vi "Keithley24XX_SR830_PPMS_4Probe_Resistance_Measurement.vi"() -> ()   [LabVIEW 2019]
uses:
  <instrlib>/Stanford Research 830/Public/Data/Read (All Parameters).vi
  <instrlib>/Keithley 24XX/Public/Data/Read (Single Point).vi
  <instrlib>/Keithley 24XX/Keithley 24XX.lvlib
  <instrlib>/Stanford Research 830/Stanford Research 830.lvlib
panel:
  in  "PPMS Temp":dbl
  out "Gate\nVoltage":sgl
  out "Status":sgl
  out "Leakage \nCurrent":sgl
  in  "Temp Vs Time":enum32{"XY Graph", "Waveform (Time)"}(tab)
  out "dup path":path
  in  "<File Name>.txt (Don't add extension)":string
  in  "Data Save Path:":path=path "C:/Users/labpc/Documents/ProbeStation Users Data"
  in  "I_leak vs Vg":enum32{"XY Graph", "Waveform (Time)"}(tab)
  out "I_leak vs Vg : XYGraph":cluster{"Y":dbl[], "Y":dbl[]}[](graph)
  out "I_leak vs Vg : TimeGraph":cluster{dbl, "Current":sgl}[](graph)
  in  "Gate Voltage\nInitial (V)":dbl
  out "Gate Voltage\nTraversal Direction":enum16{"Upward", "Downward"}(ring)
  in  "Series Resistance \n(Apparatus Constant)":dbl=10000000.0
  in  "stop":bool
  out "Max/Min(-) \nGate Voltage (V)":dbl=80.0
  in  "Gate Voltage \nStep Size (V)":dbl=0.1
  in  "High Gate \nVoltage (V)":dbl
  in  "Low Gate \nVoltage (V)":dbl
  out "Compliance\n Level (A)":dbl=0.1
  in  "Theta vs Vg":enum32{"XY Graph", "Waveform (Time)"}(tab)
  out "Theta vs Vg : XYGraph":cluster{"Y":dbl[], "Y":dbl[]}[](graph)
  out "Theta vs Vg : TimeGraph":cluster{dbl, "Theta-Value":dbl}[](graph)
  in  "R vs Vg":enum32{"XY Graph", "Waveform (Time)"}(tab)
  out "Resistance vs Vg : XYGraph":cluster{"Y":dbl[], "Y":dbl[]}[](graph)
  out "R vs Vg : TimeGraph":cluster{dbl, dbl}[](graph)
  in  "Sensitivity (Initial Value)":i16(ring)=17 items=["Auto Gain"=-1, "2 nV/fA"=0, "5 nV/fA"=1, "10 nV/fA"=2, "20 nV/fA"=3, "50 nV/fA"=4, "100 nV/fA"=5, "200 nV/fA"=6, "500 nV/fA"=7, "1 uV/pA"=8, "2 uV/pA"=9, "5 uV/pA"=10, "10 uV/pA"=11, "20 uV/pA"=12, "50 uV/pA"=13, "100 uV/pA"=14, "200 uV/pA"=15, "500 uV/pA"=16, "1 mV/nA"=17, "2 mV/nA"=18, "5 mV/nA"=19, "10 mV/nA"=20, "20 mV/nA"=21, "50 mV/nA"=22, "100 mV/nA"=23, "200 mV/nA"=24, "500 mV/mA"=25, "1 V/uA"=26]
  in  "Dynamic Reserve (-1 = Auto)":i16(ring)=-1 items=["Auto Reserve"=-1, "High Reserve"=0, "Normal"=1, "Low Noise"=2]
  in  "Input Connection (0: Single-Ended Voltage)":u16(ring)=1 items=["Single-Ended Voltage", "Differential Voltage", "1 MOhm Current Gain", "100 MOhm Current Gain"]
  out "Input Coupling (0: AC)":u16(ring) items=["AC", "DC"]
  in  "Time Constant (8: 100ms)":u16(ring)=9 items=["10 us", "30 us", "100 us", "300 us", "1 ms", "3 ms", "10 ms", "30 ms", "100 ms", "300 ms", "1 s", "3 s", "10 s", "30 s", "100 s", "300 s", "1 ks", "3 ks", "10 ks", "30 ks"]
  in  "SR830 VISA resource name":refnum<visa-resource-name>="GPIB0::10::INSTR"
  in  "Trigger Source (0: Internal)":u16(ring) items=["Internal", "External"]
  out "Manual Phase (0 Degree)":dbl
  out "Detection Harmonic Number":dbl=1.0
  out "External Reference Trigger (0: Sine Zero Crossing)":u16(ring) items=["Sine Zero Crossing", "TTL Rising Edge", "TTL Falling Edge"]
  in  "Internal Reference Frequency (1000 Hz)":dbl=17.0
  in  "Reference Source (1: Internal)":u16(ring)=1 items=["External", "Internal"]
  in  "Sine Output Amplitude (V)":dbl=1.0
  in  "Serial Configuration":T1={"Baud Rate"=9600, "Parity"=0, "Data Bits"=8, "Stop Bits"=10, "Flow Control"=0} {"Flow Control" items=["None", "XON/XOFF", "RTS/CTS", "XON/XOFF & RTS/CTS", "DTR/DSR", "XON/XOFF & DTR/DSR"]; "Stop Bits" items=["1.0"=10, "1.5"=15, "2.0"=20]; "Data Bits" items=["7"=7, "8"=8]; "Parity" items=["None", "Odd", "Even", "Mark", "Space"]; "Baud Rate" items=["300"=300, "600"=600, "1200"=1200, "2400"=2400, "4800"=4800, "9600"=9600, "19200"=19200]}
  in  "Keithley24XX VISA resource name":refnum<visa-resource-name>="GPIB0::21::INSTR" caption="Keithley 24XX VISA resource name"
  out "Interal Measurement Time":u32
  # "Lake Shore 336 Temp Contr."
  # "SR830 Lock In Amplifier"
  # "MAKE SURE THE SOURCE METER IS ON TO ENSURE NO UNINTENDED JUMPS. PROGRAM WILL KEEP SOURCE METER ON ONCE RUN."
  # "Keithley 2400 SourceMeter"
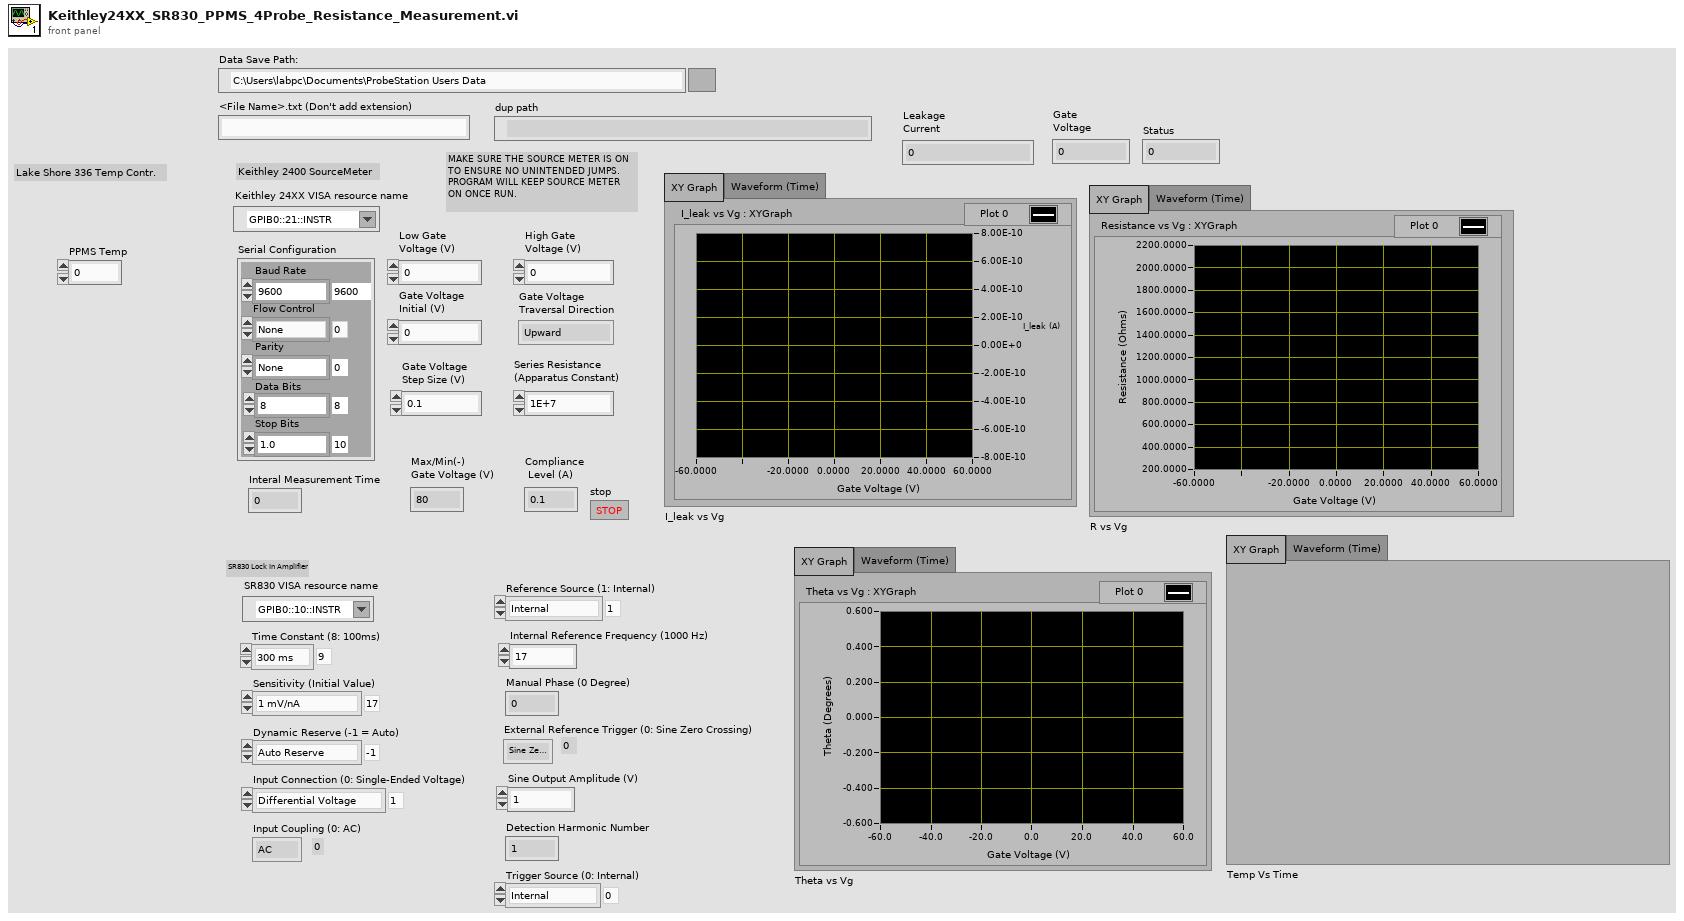
[diagram p1: front panel]
types:
  T1 = cluster{"Baud Rate":u32, "Parity":u16, "Data Bits":u16, "Stop Bits":u16, "Flow Control":u16}
  T2 = enum16{"open", "replace", "create", "open or create", "replace or create", "replace or create with confirmation"}
  T3 = cluster{"X-Value":dbl, "Y-Value":dbl, "R-Value":dbl, "Theta-Value":dbl, "Aux In 1 Value":dbl, "Aux In 2 Value":dbl, "Aux In 3 Value":dbl, "Aux In 4 Value":dbl, "Reference Frequency":dbl, "Channel 1 Display":dbl, "Channel 2 Display":dbl}
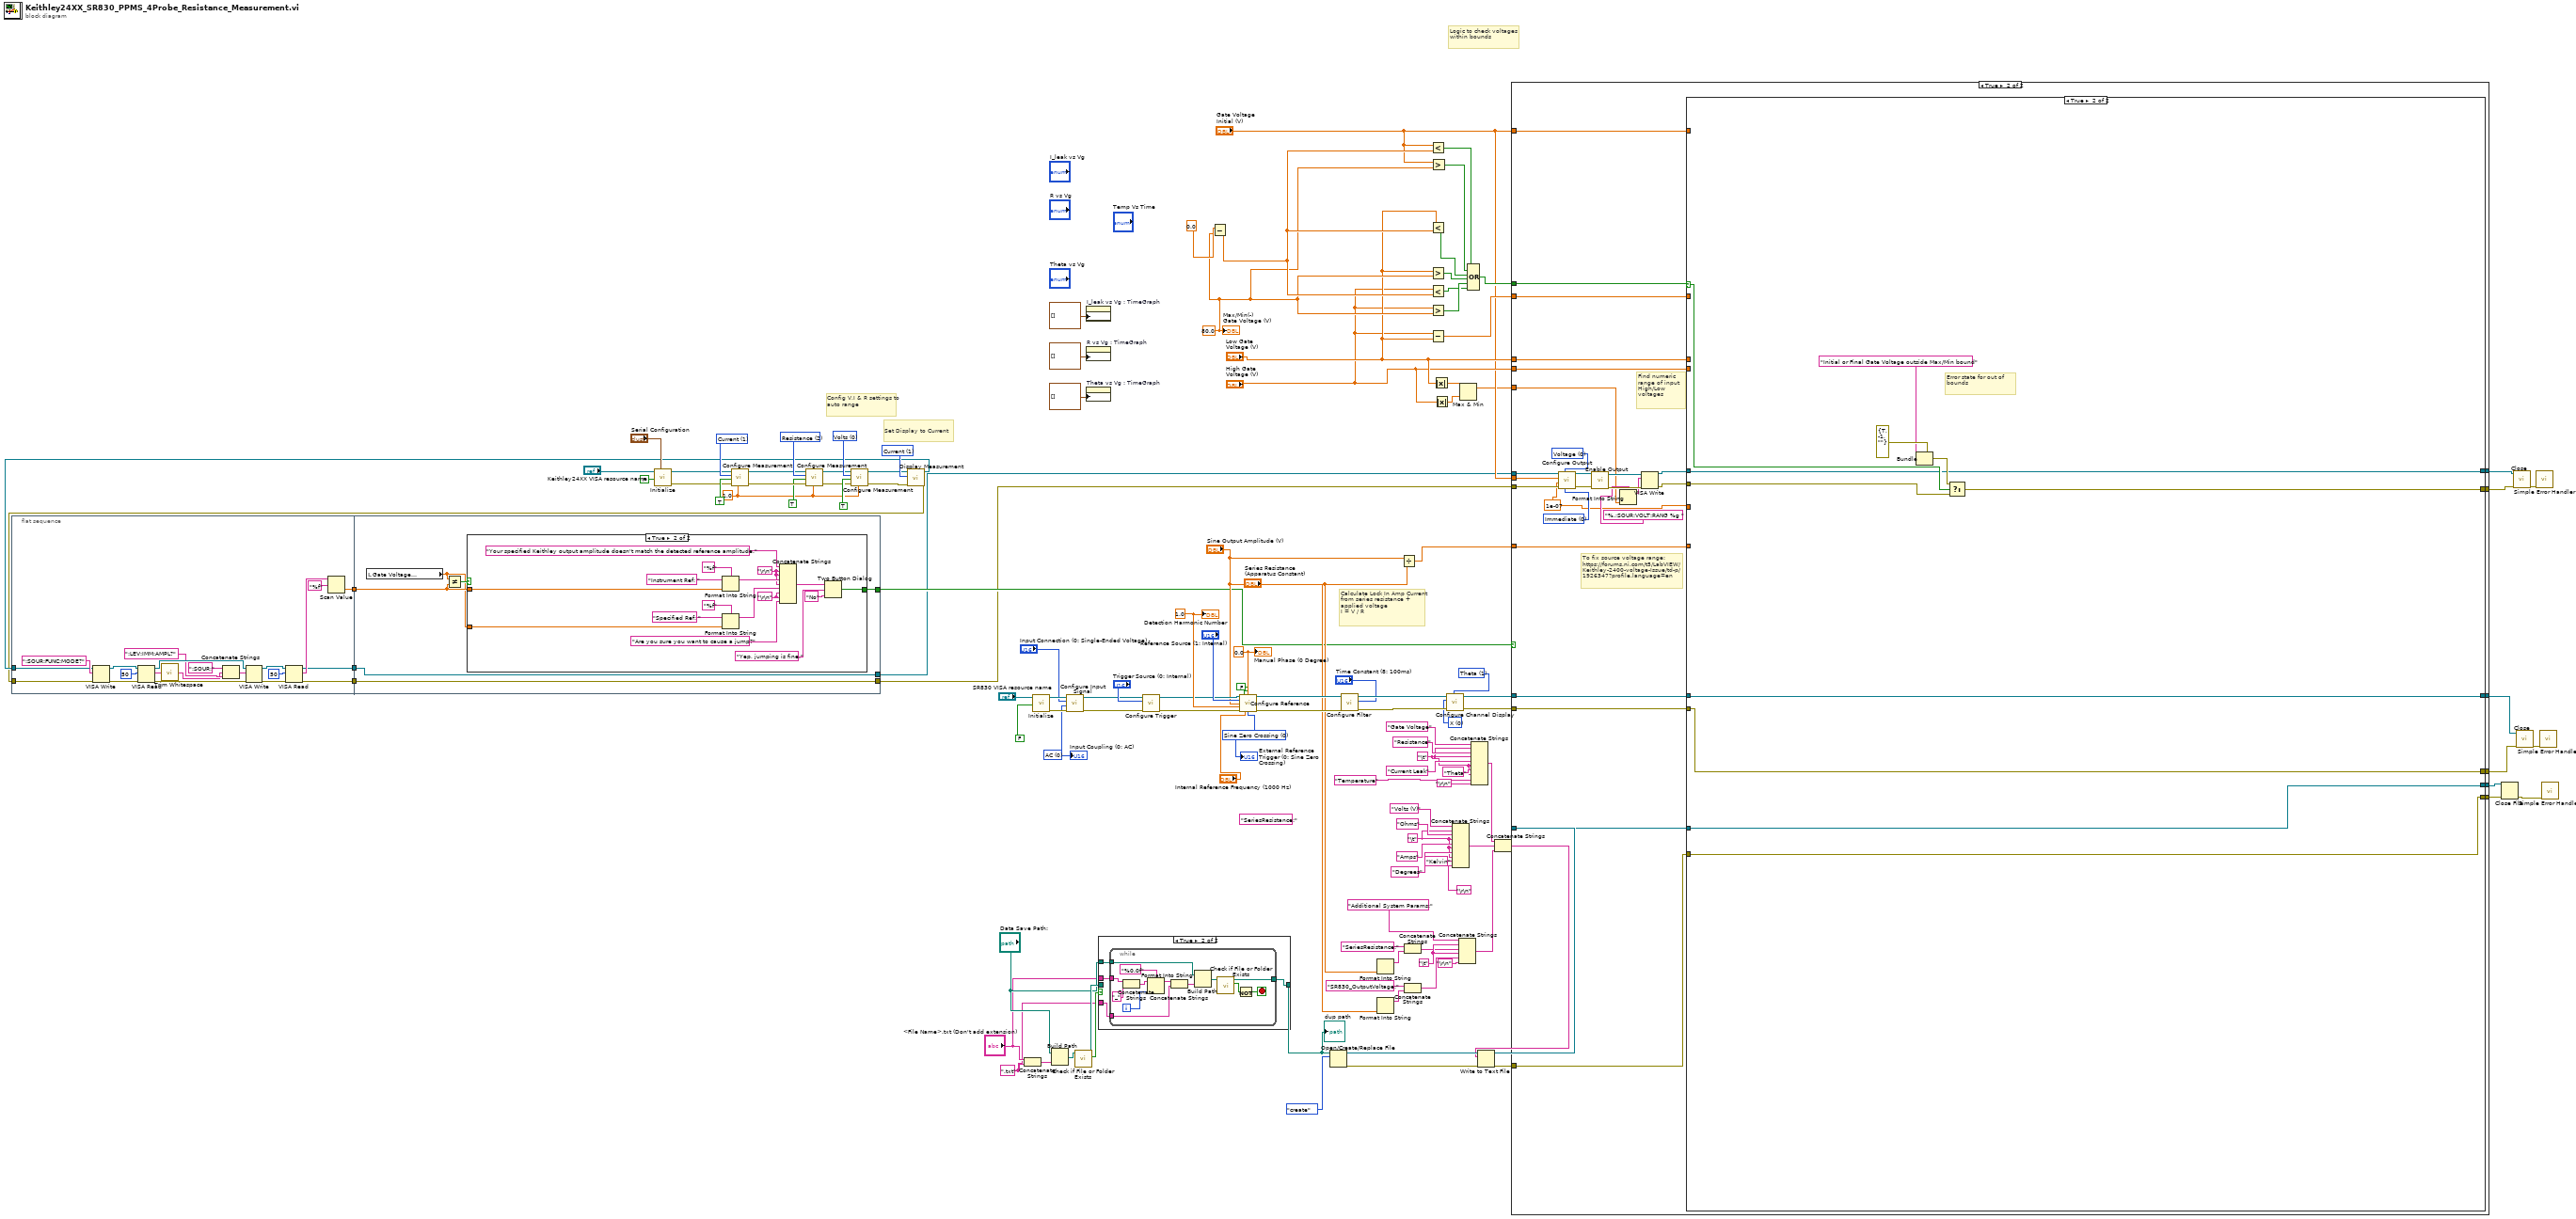
[diagram p0: block diagram]
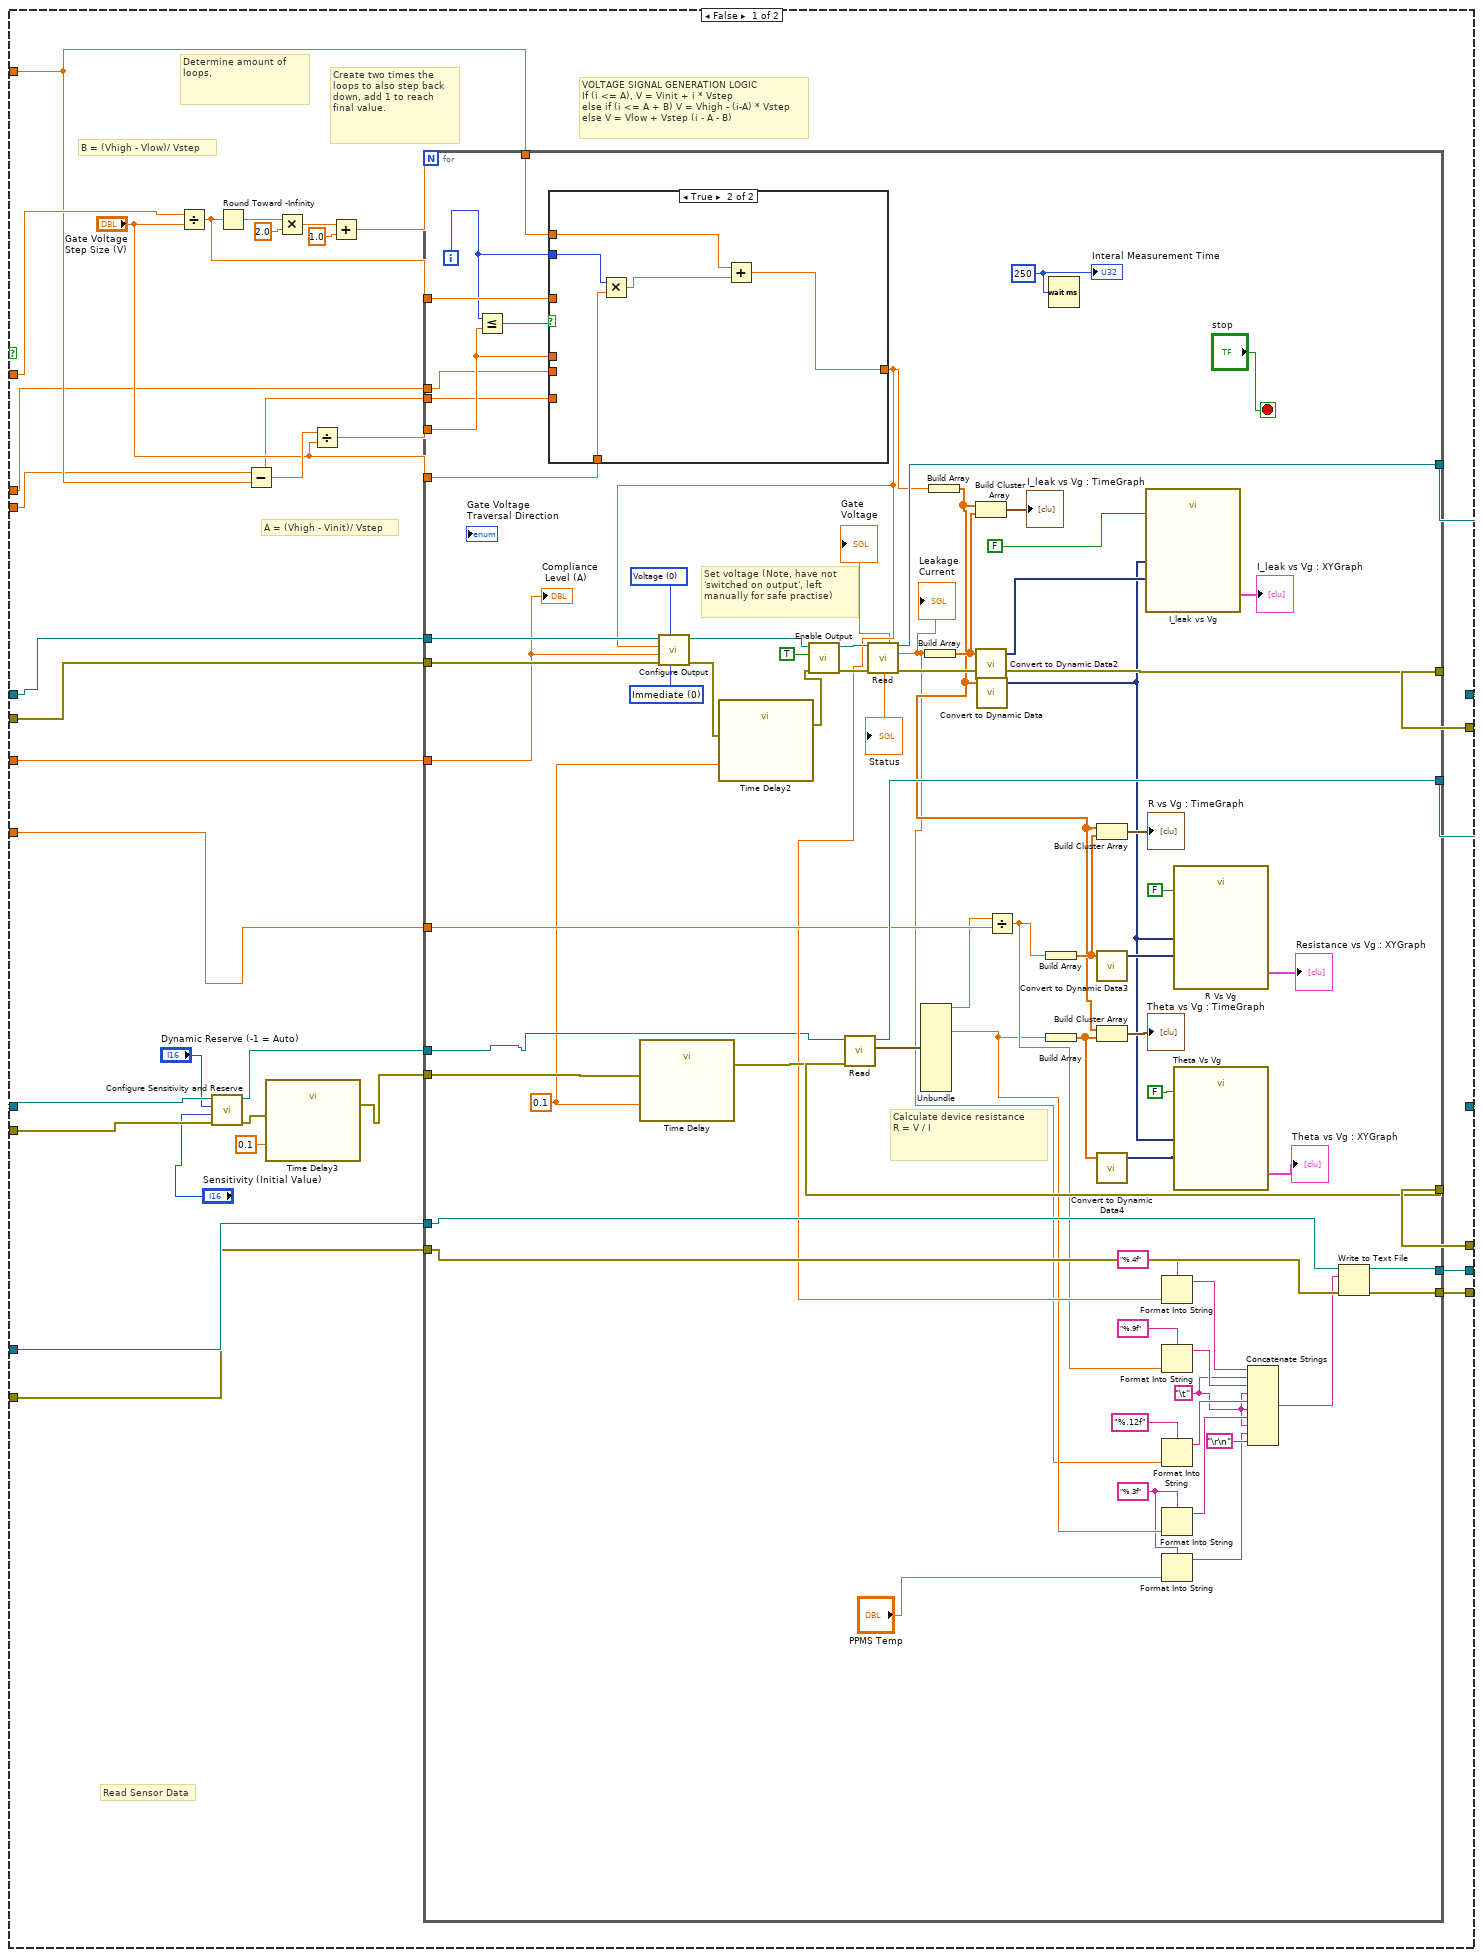
[diagram p3: hidden frame]
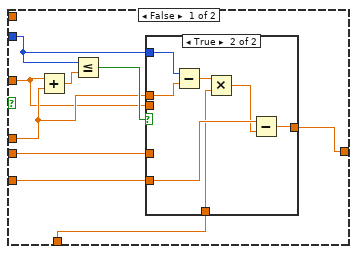
[diagram p4: hidden frame]
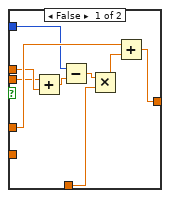
[diagram p5: hidden frame]
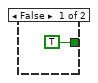
[diagram p6: hidden frame]
diagram:
  w25 = "\t"
  w16 = "\t"
  w18 = "\t"
  (unwired) "SeriesResistance:" ("string")
  w53 = ".txt"
  w60 = 1.0 ("Manual Range (1.0)")
  w84 = 0.0 ("Manual Phase (0 Degree)")
  w85 = 1.0 ("Detection Harmonic Number (1)")
  w86 = u16 0 items=["Sine Zero Crossing", "TTL Rising Edge", "TTL Falling Edge"] ("External Reference Trigger (0: Sine Zero Crossing)")
  w90 = u16 0 items=["AC", "DC"] ("Input Coupling (0: AC)")
  w72 = u16 0 items=["X", "R", "X Noise", "Aux In 1", "Aux In 2"] ("Channel 1 Display (0: X)")
  w100 = u16 1 items=["Y", "Theta", "Y Noise", "Aux In 3", "Aux In 4"] ("Channel 2 Display  (0: Y)")
  w105 = u16 1 items=["Voltage", "Current", "Resistance"] ("Displayed Measurement (0: Voltage)")
  w114 = u16 2 items=["Volts", "Current", "Resistance"] ("Function (0: Volts)")
  w118 = u16 1 items=["Volts", "Current", "Resistance"] ("Function (0: Volts)")
  w61 = 80.0
  w124 = u16 0 items=["Volts", "Current", "Resistance"] ("Function (0: Volts)")
  # "Logic to check voltages within bounds"
  # "Calculate Lock In Amp Current from series resistance + applied voltage\nI = V / R"
  # "Set Display to Current"
  # "Config V,I & R settings to auto range"
  n1 = flat-sequence {
    tunnel: [w128] -> w10
    tunnel: [w129] -> w9
    tunnel: [w130] -> w8
    tunnel: w7 -> [w127]
    tunnel: w6 -> [w126]
    tunnel: w10 -> [w149]
    tunnel: w9 -> [w148]
    tunnel: w8 -> [w152]
    tunnel: [w149] -> w2
    tunnel: [w148] -> w4
    tunnel: [w147] -> w5
    frame #0 {
      n2 = VISA Write(VISA resource name=w127, write buffer=":SOUR:FUNC:MODE?", error in (no error)=w126) -> (VISA resource name out=w143:refnum<visa-resource-name>, error out=w146:errorcluster)  [unwired: 1 out]
      n3 = VISA Read(VISA resource name=w143, byte count=u32 50, error in (no error)=w146) -> (VISA resource name out=w138:refnum<visa-resource-name>, read buffer=w132:string, error out=w139:errorcluster)  [unwired: 1 out]
      n4 = call <vilib>:"Trim Whitespace.vi"("string"=w132) -> ("trimmed string"=w131:string)  [unwired: 1 in]
      n5 = Concatenate Strings(":SOUR:" ("string"), w131, ":LEV:IMM:AMPL?" ("string")) -> (w135:string)
      n6 = VISA Write(VISA resource name=w138, write buffer=w135, error in (no error)=w139) -> (VISA resource name out=w140:refnum<visa-resource-name>, error out=w142:errorcluster)  [unwired: 1 out]
      n7 = VISA Read(VISA resource name=w140, byte count=u32 50, error in (no error)=w142) -> (VISA resource name out=w128:refnum<visa-resource-name>, read buffer=w133:string, error out=w129:errorcluster)  [unwired: 1 out]
      n8 = Scan Value(string=w133, format string="%f") -> (value=w130:dbl)  [unwired: 1 in, 1 out]
    }
    frame #1 {
      n9 = local read "Gate Voltage\nInitial (V)"() -> (w150:dbl)
      n10 = Not Equal?(x=w150, y=w152) -> (x != y?=w151:bool)
      n11 = case shown="True" w151 {
        tunnel: [TRUE ("T button?") w160] -> w147
        tunnel: w152 -> [_ w155]
        tunnel: w150 -> [_ w154]
        frame False {
        }
        frame True {
          w158 = "\r\n"
          w156 = "\r\n"
          n12 = Format Into String(format string="%f", initial string="Instrument Ref: ", w155) -> (resulting string=w162:string)  [unwired: 1 in, 1 out]
          n13 = Format Into String(format string="%f", initial string="Specified Ref: ", w154) -> (resulting string=w161:string)  [unwired: 1 in, 1 out]
          n14 = Concatenate Strings("Your specified Keithley output amplitude doesn't match the detected reference amplitude." ("message"), w156, w156, w162, w156, w161, w158, w158, "Are you sure you want to cause a jump?" ("string")) -> (w167:string)
          n15 = Two Button Dialog(message=w167, 1:"No" ("F button name (\"Cancel\")"), 2:"Yep, jumping is fine." ("T button name (\"OK\")")) -> (T button?=w160:bool)
        }
      }
    }
  }
  n16 = call <instrlib>:"Initialize.vi"("Serial Configuration"="Serial Configuration", "Reset (True)"=FALSE, "VISA resource name"="Keithley24XX VISA resource name") -> ("error out"=w109:errorcluster, "VISA resource name out"=w110:refnum<visa-resource-name>)  [unwired: 7 in]
  n17 = call <instrlib>:"Configure Measurement.vi"("Manual Range (1.0)"=w60, "error in (no error)"=w109, "Enable Auto Range (T:Enable)"=TRUE, "Function (0: Volts)"=w118, "VISA resource name"=w110) -> ("error out"=w116:errorcluster, "VISA resource name out"=w111:refnum<visa-resource-name>)  [unwired: 5 in]
  n18 = call <instrlib>:"Configure Measurement.vi"("Manual Range (1.0)"=w60, "error in (no error)"=w116, "Enable Auto Range (T:Enable)"=TRUE, "Function (0: Volts)"=w114, "VISA resource name"=w111) -> ("error out"=w113:errorcluster, "VISA resource name out"=w112:refnum<visa-resource-name>)  [unwired: 5 in]
  n19 = call <instrlib>:"Configure Measurement.vi"("Manual Range (1.0)"=w60, "error in (no error)"=w113, "Enable Auto Range (T:Enable)"=TRUE, "Function (0: Volts)"=w124, "VISA resource name"=w112) -> ("error out"=w103:errorcluster, "VISA resource name out"=w104:refnum<visa-resource-name>)  [unwired: 5 in]
  n20 = call <instrlib>:"Display Measurement.vi"("error in (no error)"=w103, "Displayed Measurement (0: Voltage)"=w105, "VISA resource name"=w104) -> ("error out"=w6:errorcluster, "VISA resource name out"=w7:refnum<visa-resource-name>)  [unwired: 7 in]
  n21 = Concatenate Strings("<File Name>.txt (Don't add extension)", w53) -> (w59:string)
  n22 = call <instrlib>:"Initialize.vi"("Reset (True)"=FALSE, "VISA resource name"="SR830 VISA resource name") -> ("error out"=w97:errorcluster, "VISA resource name out"=w98:refnum<visa-resource-name>)  [unwired: 8 in]
  n23 = Build Path(base path="Data Save Path:", name or relative path=w59) -> (appended path=w58:path)
  n24 = call <instrlib>:"Configure Input Signal.vi"("error in (no error)"=w97, "Input Coupling (0: AC)"=w90, "Input Connection (0: Single-Ended Voltage)"="Input Connection (0: Single-Ended Voltage)", "VISA resource name"=w98) -> ("error out"=w81:errorcluster, "VISA resource name out"=w82:refnum<visa-resource-name>)  [unwired: 6 in]
  n25 = call <vilib>:"Check if File or Folder Exists.vi"("path"=w58) -> ("file or folder exists?"=w57:bool, "dup path"=w56:path)  [unwired: 8 in, 1 out]
  n26 = property on="I_leak vs Vg : TimeGraph" class="WFChart (strict)"("History Data"=cluster{dbl, "Current":sgl}[] []) -> ()  [unwired: 2 in, 2 out]
  n27 = property on="R vs Vg : TimeGraph" class="WFChart (strict)"("History Data"=cluster{dbl, dbl}[] []) -> ()  [unwired: 2 in, 2 out]
  n28 = property on="Theta vs Vg : TimeGraph" class="WFChart (strict)"("History Data"=cluster{dbl, "Theta-Value":dbl}[] []) -> ()  [unwired: 2 in, 2 out]
  n29 = case shown="True" w57 {
    tunnel: [w170 w171] -> w50
    tunnel: w56 -> [w170 _]
    tunnel: "Data Save Path:" -> [_ w172]
    tunnel: "<File Name>.txt (Don't add extension)" -> [_ w174]
    tunnel: w53 -> [_ w173]
    frame False {
    }
    frame True {
      n30 = while {
        tunnel: w174 -> [w177]
        tunnel: w173 -> [w182]
        tunnel: w172 -> [w180]
        tunnel: [w178] -> w171
        i -> [w184]
        stop <- w186 stop-if-true
        n31 = Concatenate Strings(w177, "_" ("string")) -> (w176:string)
        n32 = Format Into String(format string="%0.0f", initial string=w176, w184) -> (resulting string=w183:string)  [unwired: 1 in, 1 out]
        n33 = Concatenate Strings(w183, w182) -> (w181:string)
        n34 = Build Path(base path=w180, name or relative path=w181) -> (appended path=w179:path)
        n35 = call <vilib>:"Check if File or Folder Exists.vi"("path"=w179) -> ("file or folder exists?"=w187:bool, "dup path"=w178:path)  [unwired: 8 in, 1 out]
        n36 = Not(x=w187) -> (.not. x?=w186:bool)
      }
    }
  }
  "dup path" <- w50
  n37 = call <instrlib>:"Configure Trigger.vi"("error in (no error)"=w81, "Trigger Source (0: Internal)"="Trigger Source (0: Internal)", "VISA resource name"=w82) -> ("error out"=w79:errorcluster, "VISA resource name out"=w80:refnum<visa-resource-name>)  [unwired: 7 in]
  n38 = Subtract(x=0.0, y=w61) -> (x-y=w66:dbl)
  n39 = call <instrlib>:"Configure Reference.vi"("VISA resource name"=w80, "Auto Phase (T: Enabled)"=FALSE, "Manual Phase (0 Degree)"=w84, "Reference Source (1: Internal)"="Reference Source (1: Internal)", "Sine Output Amplitude (1 V)"="Sine Output Amplitude (V)", "Detection Harmonic Number (1)"=w85, "error in (no error)"=w79, "Internal Reference Frequency (1000 Hz)"="Internal Reference Frequency (1000 Hz)", "External Reference Trigger (0: Sine Zero Crossing)"=w86) -> ("VISA resource name out"=w87:refnum<visa-resource-name>, "error out"=w88:errorcluster)  [unwired: 5 in]
  n40 = Open/Create/Replace File(file path (use dialog)=w50, operation (0:open)=T2."create") -> (refnum out=w51:refnum<file>, error out=w49:errorcluster)  [unwired: 4 in, 1 out]
  n41 = call <instrlib>:"Configure Filter.vi"("error in (no error)"=w88, "Time Constant (8: 100ms)"="Time Constant (8: 100ms)", "VISA resource name"=w87) -> ("error out"=w107:errorcluster, "VISA resource name out"=w106:refnum<visa-resource-name>)  [unwired: 7 in]
  n42 = Format Into String("Series Resistance \n(Apparatus Constant)") -> (resulting string=w43:string)  [unwired: 3 in, 1 out]
  n43 = Format Into String("Sine Output Amplitude (V)") -> (resulting string=w42:string)  [unwired: 3 in, 1 out]
  n44 = Divide(x="Sine Output Amplitude (V)", y="Series Resistance \n(Apparatus Constant)") -> (x/y=w78:dbl)
  n45 = Concatenate Strings("SeriesResistance:" ("string"), w43) -> (w24:string)
  n46 = Concatenate Strings("SR830_OutputVoltage:" ("string"), w42) -> (w23:string)
  n47 = Less?(x="Gate Voltage\nInitial (V)", y=w66) -> (x < y?=w64:bool)
  n48 = Less?(x="Low Gate \nVoltage (V)", y=w66) -> (x < y?=w70:bool)
  n49 = Greater?(x="Low Gate \nVoltage (V)", y=w61) -> (0:w69:bool)
  n50 = Less?(x="High Gate \nVoltage (V)", y=w66) -> (x < y?=w67:bool)
  n51 = Greater?(x="High Gate \nVoltage (V)", y=w61) -> (0:w68:bool)
  n52 = Subtract(x="High Gate \nVoltage (V)", y="Low Gate \nVoltage (V)") -> (x-y=w62:dbl)
  n53 = Greater?(x="Gate Voltage\nInitial (V)", y=w61) -> (0:w65:bool)
  n54 = Absolute Value(x="Low Gate \nVoltage (V)") -> (abs(x)=w14:dbl)
  n55 = Absolute Value(x="High Gate \nVoltage (V)") -> (abs(x)=w13:dbl)
  n56 = call <instrlib>:"Configure Channel Display.vi"("Channel 2 Display  (0: Y)"=w100, "error in (no error)"=w107, "Channel 1 Display (0: X)"=w72, "VISA resource name"=w106) -> ("error out"=w95:errorcluster, "VISA resource name out"=w96:refnum<visa-resource-name>)  [unwired: 6 in]
  n57 = Concatenate Strings("Volts (V)" ("string"), w16, "Ohms" ("string"), w16, "Amps" ("string"), w16, "Degrees" ("string"), w16, "Kelvin" ("string"), "\r\n") -> (w36:string)
  n58 = Concatenate Strings("Additional System Params:" ("string"), w25, w24, w25, w23, "\r\n") -> (w26:string)
  n59 = Max & Min(x=w14, y=w13) -> (max(x,y)=w1:dbl)  [unwired: 1 out]
  n60 = Compound Arithmetic op=OR(w64, w65, w70, w69, w68, w67) -> (w63:bool)
  n61 = Concatenate Strings("Gate Voltage" ("string"), w18, "Resistance" ("string"), w18, "Current Leak" ("string"), w18, "Theta" ("string"), w18, "Temperature" ("string"), "\r\n") -> (w37:string)
  n62 = Concatenate Strings(w37, w36, w26) -> (w21:string)
  n63 = Write to Text File(file (use dialog)=w51, text=w21, error in=w49) -> (refnum out=w47:refnum<file>, error out=w46:errorcluster)  [unwired: 1 in, 1 out]
  n64 = case shown="True" w5 {
    tunnel: [w193 w224] -> w122
    tunnel: [w192 w223] -> w121
    tunnel: w96 -> [w191 w222]
    tunnel: w95 -> [w190 w221]
    tunnel: [w191 w220] -> w94
    tunnel: [w190 w219] -> w93
    tunnel: w78 -> [_ w218]
    tunnel: w63 -> [_ w217]
    tunnel: w62 -> [_ w216]
    tunnel: w47 -> [w189 w215]
    tunnel: w46 -> [w188 w214]
    tunnel: [w189 w213] -> w45
    tunnel: [w188 w212] -> w44
    tunnel: "Low Gate \nVoltage (V)" -> [_ w211]
    tunnel: "High Gate \nVoltage (V)" -> [_ w210]
    tunnel: "Gate Voltage\nInitial (V)" -> [_ w209]
    tunnel: w4 -> [w192 w201]
    tunnel: "Gate Voltage\nInitial (V)" -> [_ w200]
    tunnel: w2 -> [w193 w199]
    tunnel: w1 -> [_ w197]
    frame False {
    }
    frame True {
      w203 = u16 0 items=["Immediate", "Triggered"] ("Output Type  (0: Immediate)")
      w196 = 1e-07 ("Compliance  Level (0.1)")
      w202 = u16 0 items=["Voltage", "Current"] ("Source Mode  (0: Voltage)")
      # "Find numeric range of input High/Low voltages"
      # "To fix source voltage range:\nhttps://forums.ni.com/t5/LabVIEW/Keithley-2400-voltage-Issue/td-p/1926347?profile.language=en"
      n65 = call <instrlib>:"Configure Output.vi"("Output Type  (0: Immediate)"=w203, "Source Mode  (0: Voltage)"=w202, "error in (no error)"=w201, "Compliance  Level (0.1)"=w196, "Output Level (0)"=w200, "VISA resource name"=w199) -> ("error out"=w208:errorcluster, "VISA resource name out"=w207:refnum<visa-resource-name>)  [unwired: 4 in]
      n66 = call <instrlib>:"Enable Output.vi"("error in (no error)"=w208, "VISA resource name"=w207) -> ("error out"=w206:errorcluster, "VISA resource name out"=w205:refnum<visa-resource-name>)  [unwired: 8 in]
      n67 = Format Into String(format string="%.;SOUR:VOLT:RANG %g ", w197) -> (resulting string=w204:string)  [unwired: 2 in, 1 out]
      n68 = VISA Write(VISA resource name=w205, write buffer=w204, error in (no error)=w206) -> (VISA resource name out=w194:refnum<visa-resource-name>, error out=w195:errorcluster)  [unwired: 1 out]
      n69 = case shown="True" w217 {
        selector: w217 -> [_ w370]
        tunnel: w195 -> [w257 w369]
        tunnel: w194 -> [w226 w364]
        tunnel: [w256 w364] -> w224
        tunnel: [w255 w365] -> w223
        tunnel: w222 -> [w250 w363]
        tunnel: w221 -> [w251 w362]
        tunnel: [w253 w363] -> w220
        tunnel: [w252 w362] -> w219
        tunnel: w218 -> [w247 _]
        tunnel: w216 -> [w242 _]
        tunnel: w211 -> [w235 _]
        tunnel: w210 -> [w236 _]
        tunnel: w209 -> [w238 _]
        tunnel: w215 -> [w231 w361]
        tunnel: w214 -> [w230 w360]
        tunnel: [w229 w361] -> w213
        tunnel: [w228 w360] -> w212
        tunnel: w196 -> [w225 _]
        frame False {
          # "Read Sensor Data"
          # "VOLTAGE SIGNAL GENERATION LOGIC\nIf (i <= A), V = Vinit + i * Vstep\nelse if (i <= A + B) V = Vhigh - (i-A) * Vstep\nelse V = Vlow + Vstep (i - A - B)"
          # "B = (Vhigh - Vlow)/ Vstep"
          # "A = (Vhigh - Vinit)/ Vstep"
          # "Create two times the loops to also step back down, add 1 to reach final value."
          # "Determine amount of loops,"
          n70 = Divide(x=w242, y="Gate Voltage \nStep Size (V)") -> (x/y=w237:dbl)
          n71 = call <instrlib>:"Configure Sensitivity and Reserve.vi"("error in (no error)"=w251, "Sensitivity (-1: Auto gain)"="Sensitivity (Initial Value)", "Dynamic Reserve (-1: Auto Reserve)"="Dynamic Reserve (-1 = Auto)", "VISA resource name"=w250) -> ("error out"=w233:errorcluster, "VISA resource name out"=w249:refnum<visa-resource-name>)  [unwired: 6 in]
          n72 = Round Toward -Infinity(1:w237) -> (0:w245:dbl)
          n73 = Subtract(x=w236, y=w238) -> (x-y=w241:dbl)
          n74 = call "Time Delay3"("error in (no error)"=w233, "Delay Time (s)"=0.1) -> ("error out"=w234:errorcluster)  [unwired: 9 in]
          n75 = Multiply(x=w245, y=2.0) -> (x*y=w244:dbl)
          n76 = Divide(x=w241, y="Gate Voltage \nStep Size (V)") -> (x/y=w239:dbl)
          n77 = Add(x=w244, y=1.0) -> (x+y=w243:dbl)
          n78 = for {
            N: w243 -> [_]
            tunnel: w226 -> [w325]
            tunnel: w257 -> [w290]
            tunnel: [w329] -> w256
            tunnel: [w328] -> w255
            tunnel: [w318] -> w253
            tunnel: [w319] -> w252
            tunnel: w249 -> [w271]
            tunnel: w234 -> [w272]
            tunnel: w247 -> [w316]
            tunnel: "Gate Voltage \nStep Size (V)" -> [w296]
            tunnel: w239 -> [w294]
            tunnel: w238 -> [w297]
            tunnel: w237 -> [w295]
            tunnel: w236 -> [w293]
            tunnel: w235 -> [w292]
            tunnel: w231 -> [w287]
            tunnel: w230 -> [w286]
            tunnel: [w285] -> w229
            tunnel: [w284] -> w228
            tunnel: w225 -> [w259]
            i -> [w267]
            stop <- "stop" stop-if-true
            w266 = "%.3f" ("format string")
            w264 = "\t"
            w291 = u16 0 items=["Immediate", "Triggered"] ("Output Type  (0: Immediate)")
            w270 = 0.1 ("Delay Time (s)")
            w326 = u32 250 ("milliseconds to wait")
            w321 = u16 0 items=["Voltage", "Current"] ("Source Mode  (0: Voltage)")
            # "Calculate device resistance\nR = V / I"
            # "Set voltage (Note, have not 'switched on output', left manually for safe practise)"
            n79 = Less Or Equal?(x=w267, y=w294) -> (x <= y?=w298:bool)
            n80 = case shown="True" w298 {
              tunnel: [w336 w355] -> w278
              tunnel: w297 -> [_ w358]
              tunnel: w267 -> [w333 w359]
              tunnel: w296 -> [w334 w356]
              tunnel: w295 -> [w330 _]
              tunnel: w294 -> [w332 _]
              tunnel: w293 -> [w335 _]
              tunnel: w292 -> [w331 _]
              frame False {
                n81 = Add(x=w330, y=w332) -> (x+y=w337:dbl)
                n82 = Less Or Equal?(x=w333, y=w337) -> (x <= y?=w338:bool)
                n83 = case shown="True" w338 {
                  tunnel: [w344 w353] -> w336
                  tunnel: w335 -> [_ w354]
                  tunnel: w334 -> [w346 w351]
                  tunnel: w333 -> [w341 w350]
                  tunnel: w332 -> [w340 w349]
                  tunnel: w331 -> [w347 _]
                  tunnel: w330 -> [w339 _]
                  frame False {
                    n84 = Add(x=w339, y=w340) -> (x+y=w342:dbl)
                    n85 = Subtract(x=w341, y=w342) -> (x-y=w343:dbl)
                    n86 = Multiply(x=w343, y=w346) -> (x*y=w345:dbl)
                    n87 = Add(x=w347, y=w345) -> (x+y=w344:dbl)
                  }
                  frame True {
                    n88 = Subtract(x=w350, y=w349) -> (x-y=w352:dbl)
                    n89 = Multiply(x=w352, y=w351) -> (x*y=w348:dbl)
                    n90 = Subtract(x=w354, y=w348) -> (x-y=w353:dbl)
                  }
                }
              }
              frame True {
                n91 = Multiply(x=w359, y=w356) -> (x*y=w357:dbl)
                n92 = Add(x=w358, y=w357) -> (x+y=w355:dbl)
              }
            }
            n93 = call "Time Delay"("error in (no error)"=w272, "Delay Time (s)"=w270) -> ("error out"=w314:errorcluster)  [unwired: 9 in]
            n94 = call <instrlib>:"Configure Output.vi"("Output Type  (0: Immediate)"=w291, "Source Mode  (0: Voltage)"=w321, "error in (no error)"=w290, "Compliance  Level (0.1)"=w259, "Output Level (0)"=w278, "VISA resource name"=w325) -> ("error out"=w289:errorcluster, "VISA resource name out"=w324:refnum<visa-resource-name>)  [unwired: 4 in]
            n95 = call "Time Delay2"("error in (no error)"=w289, "Delay Time (s)"=w270) -> ("error out"=w288:errorcluster)  [unwired: 9 in]
            n96 = call <instrlib>:"Enable Output.vi"("error in (no error)"=w288, "Enable Output (T: Enable)"=TRUE, "VISA resource name"=w324) -> ("error out"=w323:errorcluster, "VISA resource name out"=w322:refnum<visa-resource-name>)  [unwired: 7 in]
            n97 = call-poly <instrlib>:"Read.vi"("error in (no error)"=w314, "VISA resource name"=w271) -> ("error out"=w319:errorcluster, "Parameter Values"=w317:T3, "VISA resource name out"=w318:refnum<visa-resource-name>)  [unwired: 7 in]
            n98 = call-poly <instrlib>:"Read.vi"("VISA resource name"=w322, "error in (no error)"=w323) -> ("Voltage"=→"Gate\nVoltage":sgl, "VISA resource name out"=w329:refnum<visa-resource-name>, "Current"=w262:sgl, "Status"=→"Status":sgl, "error out"=w328:errorcluster)  [unwired: 7 in, 2 out]
            "Leakage \nCurrent" <- w262
            n99 = Unbundle(w317) -> ("X-Value"=w315:dbl, "Theta-Value"=w276:dbl)  [unwired: 9 out]
            n100 = Build Array(w262) -> (w311:sgl[])
            n101 = Build Array(w278) -> (w269:dbl[])
            n102 = Build Cluster Array(w269, w311) -> (→"I_leak vs Vg : TimeGraph":cluster{dbl, "Current":sgl}[])
            n103 = call "Convert to Dynamic Data2"("Array"=w311) -> ("Dynamic Data Type"=w310:dynamicdata)  [unwired: 3 in]
            n104 = call "Convert to Dynamic Data"("Array"=w269) -> ("Dynamic Data Type"=w268:dynamicdata)  [unwired: 3 in]
            n105 = Divide(x=w315, y=w316) -> (x/y=w277:dbl)
            n106 = Build Array(w277) -> (w309:dbl[])
            n107 = Build Array(w276) -> (w307:dbl[])
            n108 = Wait (ms)(milliseconds to wait=w326) -> ()  [unwired: 1 out]
            n109 = Build Cluster Array(w269, w309) -> (→"R vs Vg : TimeGraph":cluster{dbl, dbl}[])
            n110 = call "Convert to Dynamic Data3"("Array"=w309) -> ("Dynamic Data Type"=w308:dynamicdata)  [unwired: 3 in]
            n111 = Build Cluster Array(w269, w307) -> (→"Theta vs Vg : TimeGraph":cluster{dbl, "Theta-Value":dbl}[])
            n112 = call "Convert to Dynamic Data4"("Array"=w307) -> ("Dynamic Data Type"=w306:dynamicdata)  [unwired: 3 in]
            n113 = call "I_leak vs Vg"("Reset"=FALSE, "Y Input"=w310, "X Input"=w268) -> ("XY Graph"=→"I_leak vs Vg : XYGraph":cluster{"X":dbl[], "Y":dbl[]}[])  [unwired: 7 in, 1 out]
            n114 = Format Into String(format string="%.4f", w278) -> (resulting string=w283:string)  [unwired: 2 in, 1 out]
            n115 = Format Into String(format string="%.9f", w277) -> (resulting string=w282:string)  [unwired: 2 in, 1 out]
            n116 = Format Into String(format string="%.12f", w262) -> (resulting string=w281:string)  [unwired: 2 in, 1 out]
            n117 = Format Into String(format string=w266, w276) -> (resulting string=w280:string)  [unwired: 2 in, 1 out]
            n118 = Format Into String(format string=w266, "PPMS Temp") -> (resulting string=w263:string)  [unwired: 2 in, 1 out]
            n119 = call "R Vs Vg"("Reset"=FALSE, "Y Input"=w308, "X Input"=w268) -> ("XY Graph"=→"Resistance vs Vg : XYGraph":cluster{"X":dbl[], "Y":dbl[]}[])  [unwired: 7 in, 1 out]
            n120 = call "Theta Vs Vg"("Reset"=FALSE, "Y Input"=w306, "X Input"=w268) -> ("XY Graph"=→"Theta vs Vg : XYGraph":cluster{"X":dbl[], "Y":dbl[]}[])  [unwired: 7 in, 1 out]
            n121 = Concatenate Strings(w283, w264, w282, w264, w281, w264, w280, w264, w263, "\r\n") -> (w279:string)
            n122 = Write to Text File(file (use dialog)=w287, text=w279, error in=w286) -> (refnum out=w285:refnum<file>, error out=w284:errorcluster)  [unwired: 1 in, 1 out]
            "Compliance\n Level (A)" <- w259
            "Interal Measurement Time" <- w326
          }
        }
        frame True {
          # "Error state for out of bounds"
          n123 = Bundle(cluster=errorcluster {"status"=TRUE, "code"=-1, "source"=""} ("error constant"), "source"="Initial or Final Gate Voltage outside Max/Min bound") -> (w366:errorcluster)  [unwired: 2 in]
          n124 = Select(t=w366, s=w370, f=w369) -> (s? t:f=w365:errorcluster)
        }
      }
    }
  }
  n125 = Close File(refnum=w45, error in=w44) -> (error out=w48:errorcluster)  [unwired: 1 out]
  n126 = call <instrlib>:"Close.vi"("error in (no error)"=w121, "VISA resource name"=w122) -> ("error out"=w120:errorcluster)  [unwired: 9 in]
  n127 = call <instrlib>:"Close.vi"("error in (no error)"=w93, "VISA resource name"=w94) -> ("error out"=w108:errorcluster)  [unwired: 9 in]
  n128 = call <vilib>:"Simple Error Handler.vi"("error in (no error)"=w120) -> ()  [unwired: 4 in, 5 out]
  n129 = call <vilib>:"Simple Error Handler.vi"("error in (no error)"=w108) -> ()  [unwired: 4 in, 5 out]
  n130 = call <vilib>:"Simple Error Handler.vi"("error in (no error)"=w48) -> ()  [unwired: 4 in, 5 out]
  "Max/Min(-) \nGate Voltage (V)" <- w61
  "Input Coupling (0: AC)" <- w90
  "External Reference Trigger (0: Sine Zero Crossing)" <- w86
  "Detection Harmonic Number" <- w85
  "Manual Phase (0 Degree)" <- w84
